vi "General Deposition Low Level Write.vi"(8 "Error In":errorcluster, 9 "Current Layer ID":i32, 10 "Layer Information Cluster":T2 {"Deposition Method" items=["Blade Coating", "Spin Coating", "Thermal Evaporation", "E-Beam Evaporation", "Sputtering", "Drop Casting", "Dip Coating", "Pulsed Laser Deposition", "Chemival Vapour Deposition", "Atomic Layer Deposition", "Spray Coating", "Screen Printing", "Electroplating", "Molecular Beam Epitaxy", "Custom Deposition"]; "Layer Type" items=["Front Electrode", "Electron Transport Layer", "Active Layer", "Hole Transport Layer", "Back Electrode", "Custom Layer"]}, 11 "Refnum in":T1) -> (0 "Error Out":errorcluster, 3 "Refnum out":T1)   [LabVIEW 2020]
uses:
  Data Clusters/Layer Information Cluster.ctl
  <vilib>/addons/database/Connection.llb/Conn ObjectReference.ctl
  <vilib>/addons/database/NI_Database_API.lvlib
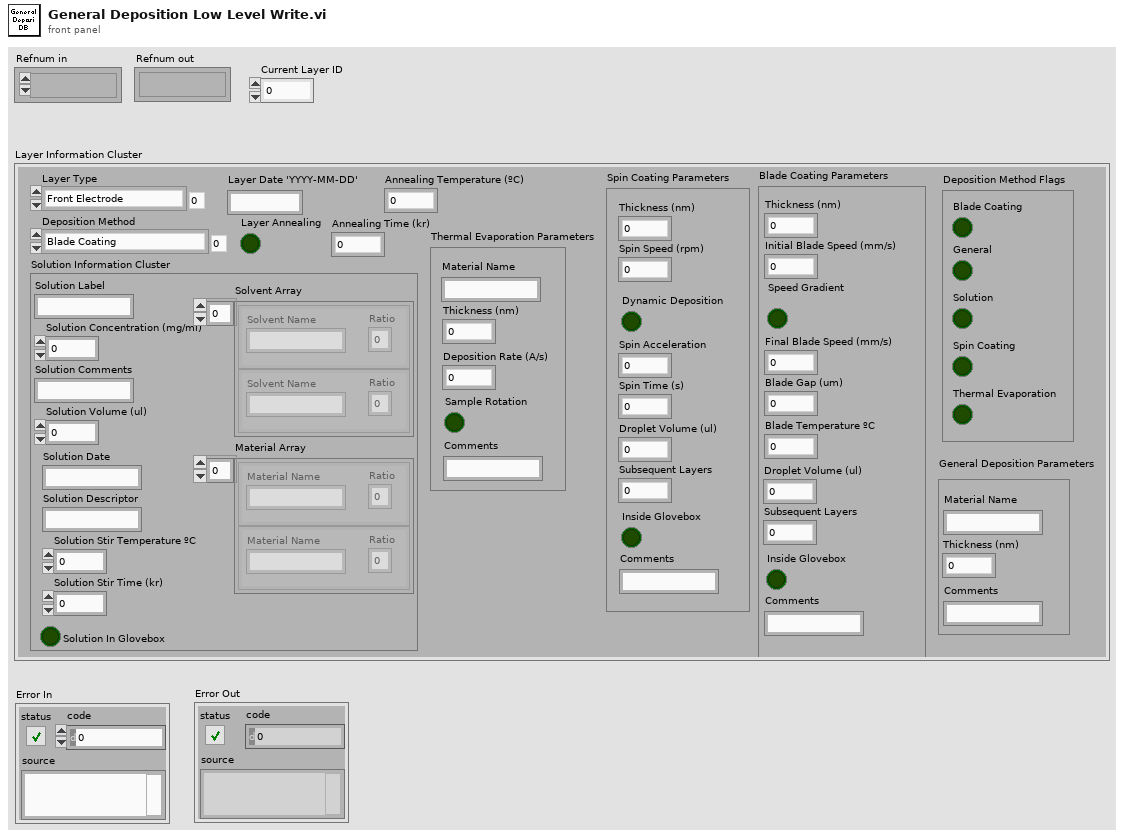
[diagram p1: front panel]
types:
  T1 = typedef "NI_Database_API.lvlib/Conn ObjectReference.ctl" = refnum<k1>
  T2 = typedef "Layer Information Cluster.ctl" = cluster{"Solution Information Cluster":cluster{"Solution Label":string, "Solution Concentration (mg/ml)":dbl, "Solution Comments ":string, "Solution Volume (ul) ":dbl, "Solution Date ":string, "Solution Descriptor ":string, "Solution Stir Temperature ºC ":dbl, "Solution Stir Time (kr) ":dbl, "Solution In Glovebox":bool, "Solvent Array":cluster{"Solvent Name":string, "Ratio":dbl}[], "Material Array":cluster{"Material Name":string, "Ratio":dbl}[]}, "Layer Type":u16, "Deposition Method":u16, "Layer Annealing":bool, "General Deposition Parameters":cluster{"Thickness (nm)":dbl, "Comments":string, "Material Name":string}, "Blade Coating Parameters":cluster{"Thickness (nm)":dbl, "Initial Blade Speed (mm/s)":dbl, "Speed Gradient":bool, "Final Blade Speed (mm/s)":dbl, "Blade Gap (um)":dbl, "Droplet Volume (ul)":dbl, "Subsequent Layers":dbl, "Inside Glovebox":bool, "Comments":string, "Blade Temperature ºC":dbl}, "Spin Coating Parameters":cluster{"Thickness (nm)":dbl, "Spin Speed (rpm)":dbl, "Dynamic Deposition":bool, "Spin Acceleration":dbl, "Spin Time (s)":dbl, "Droplet Volume (ul)":dbl, "Subsequent Layers":dbl, "Inside Glovebox":bool, "Comments":string}, "Thermal Evaporation Parameters":cluster{"Deposition Rate (A/s)":dbl, "Thickness (nm)":dbl, "Comments":string, "Material Name":string, "Sample Rotation":bool}, "Layer Date 'YYYY-MM-DD'":string, "Annealing Time (kr)":dbl, "Annealing Temperature (ºC)":dbl, "Deposition Method Flags":cluster{"Blade Coating":bool, "General ":bool, "Solution":bool, "Spin Coating":bool, "Thermal Evaporation":bool}}
  T3 = cluster{"Material Name":string, "Thickness (nm)":dbl, "Comments":string, "Current Layer ID":i32}
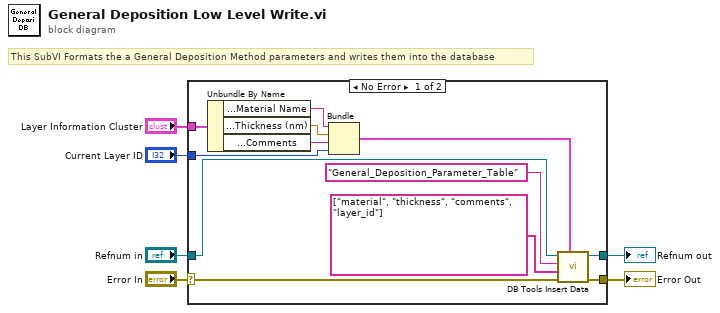
[diagram p0: block diagram]
diagram:
  # "This SubVI Formats the a General Deposition Method parameters and writes them into the database"
  n1 = case shown="No Error" "Error In" {
    selector: "Error In" -> [w17 w19]
    tunnel: "Layer Information Cluster" -> [w18 _]
    tunnel: "Current Layer ID" -> [w7 _]
    tunnel: "Refnum in" -> [w16 w20]
    tunnel: [w15 w20] -> w2
    tunnel: [w14 w19] -> w1
    frame No Error {
      n2 = Unbundle By Name(w18) -> ("General Deposition Parameters.Material Name"=w10:string, "General Deposition Parameters.Thickness (nm)"=w9:dbl, "General Deposition Parameters.Comments"=w8:string)
      n3 = Bundle("Material Name"=w10, "Thickness (nm)"=w9, "Comments"=w8, "Current Layer ID"=w7) -> (w11:T3)  [unwired: 1 in]
      n4 = call <vilib>:"DB Tools Insert Data.vi"("data"=w11, "error in (no error)"=w17, "columns"=string[] ["material", "thickness", "comments", "layer_id"], "table"="General_Deposition_Parameter_Table", "connection reference"=w16) -> ("error out"=w14:errorcluster, "connection reference out"=w15:T1)  [unwired: 5 in]
    }
    frame Error {
    }
  }
  "Refnum out" <- w2
  "Error Out" <- w1
